vi "Sort Chat[ ].vi"(8 "error in (no error)":errorcluster, 11 "Telegram Class in":refnum<class "Telegram Class.lvclass">) -> (0 "error out":errorcluster, 3 "Telegram Class out":refnum<class "Telegram Class.lvclass">)   [LabVIEW 2015, in "Telegram Library.lvlib" / "Telegram Class.lvclass"]
doc: "Created IvanLis by LabVIEW Portal\nProfile: http://labviewportal.org/memberlist.php?mode=viewprofile&u=987\neMail: IvanLisanov@gMail.com\nTelegram: https://t.me/IvanLis"
uses:
  Telegram Class.lvclass
  Telegram Class.lvclass/Telegram Class.ctl
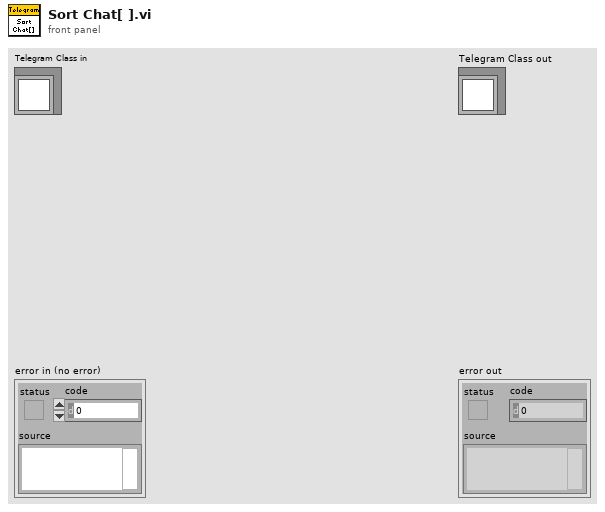
[diagram p1: front panel]
types:
  T1 = typedef "Telegram Library.lvlib/Chat.ctl" = cluster{"id":i64, "position":i64, "title":string}
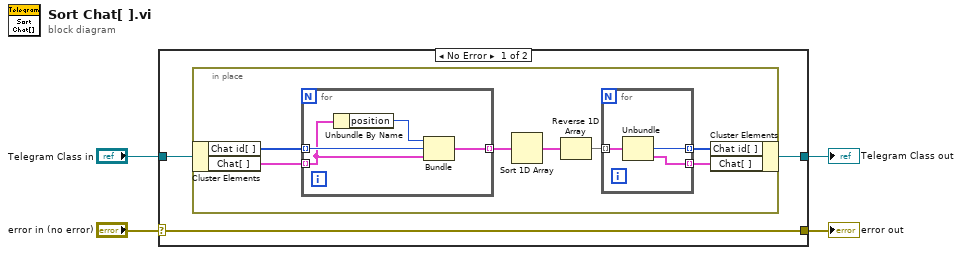
[diagram p0: block diagram]
diagram:
  n1 = case shown="No Error" "error in (no error)" {
    selector: "error in (no error)" -> [w7 w23]
    tunnel: [w7 w23] -> w3
    tunnel: [w5 w22] -> w1
    tunnel: "Telegram Class in" -> [w6 w22]
    frame No Error {
      n2 = in-place {
        n3 = in-place-cluster #1(w6) -> ("Chat id[ ]"=w14:i64[], "Chat[ ]"=w13:T1[])
        n4 = for {
          tunnel: w14 -> [w18] mode=indexing
          tunnel: w13 -> [w16] mode=indexing
          tunnel: [w17] -> w12 mode=indexing
          n5 = Unbundle By Name(w16) -> ("position"=w15:i64)
          n6 = Bundle("position"=w15, "id"=w18, "Chat"=w16) -> (w17:cluster{"position":i64, "id":i64, "Chat":T1})  [unwired: 1 in]
        }
        n7 = Sort 1D Array(array=w12) -> (sorted array=w11:cluster{"position":i64, "id":i64, "Chat":T1}[])
        n8 = Reverse 1D Array(array=w11) -> (reversed array=w8:cluster{"position":i64, "id":i64, "Chat":T1}[])
        n9 = for {
          tunnel: w8 -> [w21] mode=indexing
          tunnel: [w20] -> w10 mode=indexing
          tunnel: [w19] -> w9 mode=indexing
          n10 = Unbundle(w21) -> ("id"=w20:i64, "Chat"=w19:T1)  [unwired: 1 out]
        }
        n11 = in-place-cluster #1("Chat id[ ]"=w10, "Chat[ ]"=w9) -> (w5:refnum<class "Telegram Class.lvclass">)
      }
    }
    frame Error {
    }
  }
  "error out" <- w3
  "Telegram Class out" <- w1
